vi "nicrio_Mdk2Api_WaitOnDone.vi"(2 "Comm Core I/O References":T1={"Command Interface"="Mod1/Command Interface", "Configuration Interface"="Mod1/Configuration Interface", "Debug Interface"="Mod1/Debug Interface", "Timing Interface"="Mod1/Timing Interface", "Status Interface"="Mod1/Status Interface", "DIO(7:0)"="Mod1/DIO(7:0)", "DIO0"="Mod1/DIO0", "DIO1"="Mod1/DIO1", "DIO2"="Mod1/DIO2", "DIO3"="Mod1/DIO3", "DIO4"="Mod1/DIO4", "DIO5"="Mod1/DIO5", "DIO6"="Mod1/DIO6", "DIO7"="Mod1/DIO7", "DIO8"="Mod1/DIO8"}) -> (4 "Timed Out?":bool)   [LabVIEW 2017]
uses:
  <vilib>/LabVIEW Targets/FPGA/cRIO/shared/nicrio_Mdk2Api/nicrio_Mdk2Api_IOReferences.ctl
  <vilib>/rvi/eio/common/nirviEmuTemplateMethod_errors.vi
  <vilib>/eio/EIOMethodNode/EIOMethodNode.xnode
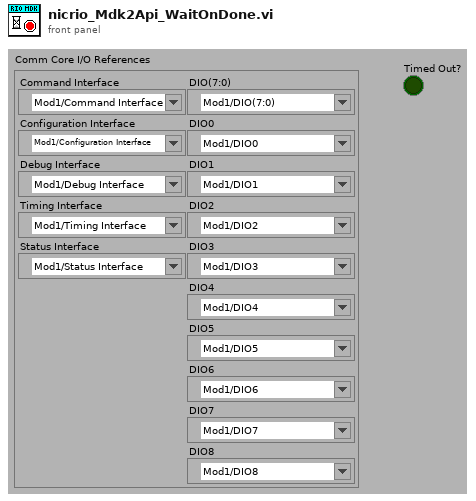
[diagram p1: front panel]
types:
  T1 = typedef "nicrio_Mdk2Api_IOReferences.ctl" = cluster{"Command Interface":refnum<k21>, "Configuration Interface":refnum<k21>, "Debug Interface":refnum<k21>, "Timing Interface":refnum<k21>, "Status Interface":refnum<k21>, "DIO(7:0)":refnum<k21>, "DIO0":refnum<k21>, "DIO1":refnum<k21>, "DIO2":refnum<k21>, "DIO3":refnum<k21>, "DIO4":refnum<k21>, "DIO5":refnum<k21>, "DIO6":refnum<k21>, "DIO7":refnum<k21>, "DIO8":refnum<k21>}
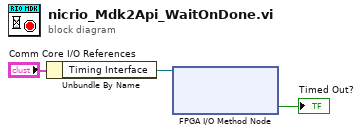
[diagram p0: block diagram]
diagram:
  n1 = Unbundle By Name("Comm Core I/O References") -> ("Timing Interface"=w2:refnum<k21>)
  n2 = xnode "FPGA I/O Method Node"("FPGA I/O In"=w2) -> ("Timed Out?"=→"Timed Out?":bool)  [unwired: 1 out]
